vi "Create Transfer Groups.vi"(8 "error in (no error)":errorcluster, 10 "Transfer Group Configurations":T1[](array[typedef]) {"Transfers"."channel configurations"."buffer offset" format="%d bytes"}, 11 "Framework in":refnum<class "Framework.lvclass">) -> (0 "error out":errorcluster, 2 "Transfer Groups":refnum<class "Transfer Group.lvclass">[](array[class]), 3 "Framework out":refnum<class "Framework.lvclass">)   [LabVIEW 2017, in "DSF Core.lvlib" / "Framework.lvclass"]
uses:
  Framework.lvclass
  Transfer Group/Transfer Group.lvclass
  Configuration/Public/Controls/DSF Engine Transfer Group Configuration.ctl
  Configuration/Public/Controls/DSF Direction.ctl
  Configuration/Public/Controls/DSF Timing Info.ctl
  Configuration/Public/Controls/DSF Engine Transfer Configuration.ctl
  Configuration/Public/Controls/DSF Byte Order.ctl
  Configuration/Public/Controls/DSF Engine Channel Configuration.ctl
  Configuration/Public/Controls/DSF Data Type.ctl
  Configuration/Public/Controls/DSF Settings Info.ctl
  Framework.lvclass/Framework.ctl
  Cache/Cache.lvclass/Cache.ctl
  Pointer/DBL Pointer.lvclass
  C:/Program Files (x86)/National Instruments/LabVIEW 2017/vi.lib/NI/Memory Manager/Classes/Pointer/Pointer.lvclass
  <vilib>/NI/Memory Manager/Classes/Pointer/Pointer.lvclass/Pointer.ctl
  <vilib>/NI/Memory Manager/Classes/Pointer/Public/New/New (8B).vi
  <vilib>/NI/Memory Manager/Classes/Pointer/Private/Allocate.vi
  <vilib>/NI/Memory Manager/Classes/Pointer/API/Accessors/Set Address.vi
  <vilib>/NI/Memory Manager/Classes/Pointer/API/Accessors/Set Size.vi
  <vilib>/NI/Memory Manager/Classes/Pointer/Private/Set Internal.vi
  Timing/Timing.lvclass
  Cache/Cache.lvclass
  DSF Core.lvlib
  Buffer/Buffer.lvclass
  <vilib>/NI/Memory Manager/Classes/Pointer/Pointer.lvclass
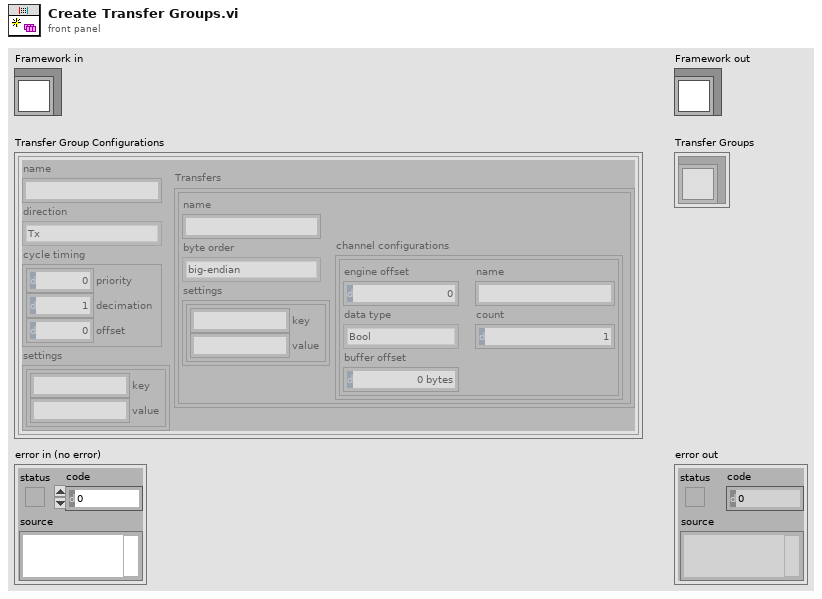
[diagram p1: front panel]
types:
  T1 = typedef "DSF Core.lvlib/DSF Engine Transfer Group Configuration.ctl" = cluster{"name":string, "direction":T2, "cycle timing":T3, "Transfers":T4[], "settings":T8}
  T2 = typedef "DSF Core.lvlib/DSF Direction.ctl" = enum8{"Tx", "Rx"}
  T3 = typedef "DSF Core.lvlib/DSF Timing Info.ctl" = cluster{"priority":u64, "decimation":u64, "offset":u64}
  T4 = typedef "DSF Core.lvlib/DSF Engine Transfer Configuration.ctl" = cluster{"name":string, "byte order":T5, "channel configurations":T6[], "settings":T8}
  T5 = typedef "DSF Core.lvlib/DSF Byte Order.ctl" = enum8{"big-endian", "little-endian"}
  T6 = typedef "DSF Core.lvlib/DSF Engine Channel Configuration.ctl" = cluster{"engine offset":u64, "name":string, "data type":T7, "count":u64, "buffer offset":u64}
  T7 = typedef "DSF Core.lvlib/DSF Data Type.ctl" = enum8{"Bool", "SGL", "DBL", "I8", "I16", "I32", "I64", "U8", "U16", "U32", "U64"}
  T8 = typedef "DSF Core.lvlib/DSF Settings Info.ctl" = cluster{"key":string, "value":string}[]
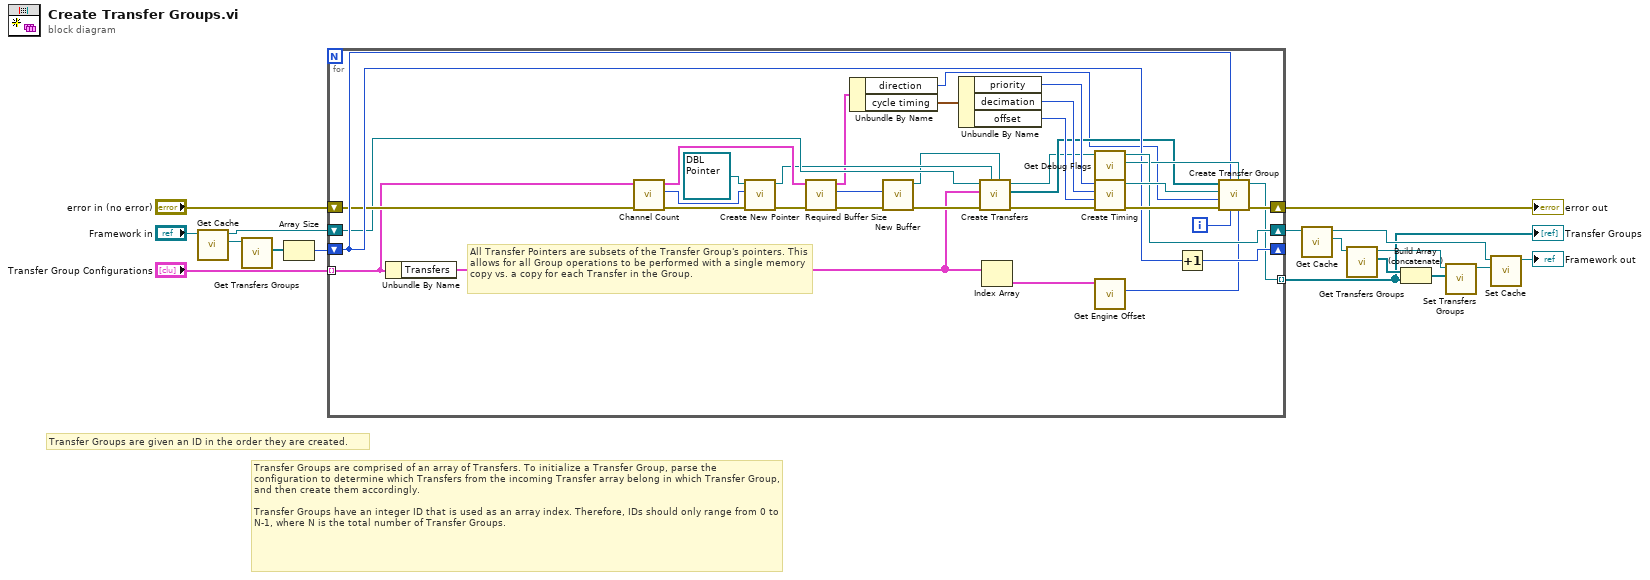
[diagram p0: block diagram]
diagram:
  # "Transfer Groups are given an ID in the order they are created."
  # "Transfer Groups are comprised of an array of Transfers. To initialize a Transfer Group, parse the configuration to determine which Transfers from the incoming Transfer array belong in which Transfer Group, and then create them accordingly.\n\nTransfer Groups have an integer ID that is used as an array index. Therefore, IDs should only range from 0 to N-1, where N is the total number of Transfer Groups."
  n1 = call "Get Cache.vi"("Framework in"="Framework in") -> ("Cache"=w6:refnum<class "Cache.lvclass">, "Framework out"=w4:refnum<class "Framework.lvclass">)  [unwired: 9 in]
  n2 = call "Get Transfers Groups.vi"("Cache in"=w6) -> ("Transfers Groups"=w3:refnum<class "Transfer Group.lvclass">[])  [unwired: 9 in, 1 out]
  n3 = Array Size(array=w3) -> (size(s)=w16:i32)
  n4 = for {
    shift-right: [w51] -> w1
    shift-left: "error in (no error)" -> [w39]
    tunnel: [w40] -> w2 mode=indexing
    shift-right: [w44] -> w8
    shift-left: w4 -> [w31]
    shift-right: [w50] -> _
    shift-left: w16 -> [w42]
    tunnel: "Transfer Group Configurations" -> [w23] mode=indexing
    i -> [w41]
    # "All Transfer Pointers are subsets of the Transfer Group's pointers. This allows for all Group operations to be performed with a single memory copy vs. a copy for each Transfer in the Group."
    n5 = Unbundle By Name(w23) -> ("Transfers"=w22:T4[])
    n6 = call "Channel Count.vi"("error in (no error)"=w39, "Transfer Group Configuration in"=w23) -> ("error out"=w29:errorcluster, "total channel count"=w24:u64, "Transfer Group Configuration out"=w38:T1)  [unwired: 7 in]
    n7 = call-poly <vilib>:"Create New Pointer.vi"("error in (no error)"=w29, "count (1)"=w24, "Pointer type"=refnum<class "DBL Pointer.lvclass"> refnum ("Group Intermediate Buffer")) -> ("error out"=w28:errorcluster, "Pointer"=w27:refnum<class "DBL Pointer.lvclass">)  [unwired: 7 in]
    n8 = call "Required Buffer Size.vi"("error in (no error)"=w28, "Transfer Group Configuration in"=w38) -> ("error out"=w36:errorcluster, "required buffer size"=w37:u64, "Transfer Group Configuration out"=w20:T1)  [unwired: 7 in]
    n9 = Unbundle By Name(w20) -> ("direction"=w19:T2, "cycle timing"=w18:T3)
    n10 = call "New Buffer.vi"("error in (no error)"=w36, "size"=w37) -> ("error out"=w35:errorcluster, "Buffer out"=w26:refnum<class "Buffer.lvclass">)  [unwired: 8 in]
    n11 = Unbundle By Name(w18) -> ("priority"=w46:u64, "decimation"=w47:u64, "offset"=w48:u64)
    n12 = call "Create Transfers.vi"("Group String Buffer"=w26, "Group Intermediate Buffer"=w27, "error in (no error)"=w35, "Transfer Configurations"=w22, "Framework in"=w31) -> ("error out"=w34:errorcluster, "Transfers"=w33:refnum<class "Transfer.lvclass">[], "Framework out"=w32:refnum<class "Framework.lvclass">)  [unwired: 4 in]
    n13 = Index Array(array=w22) -> (element=w21:T4)  [unwired: 1 in]
    n14 = call "Get Debug Flags.vi"("Framework in"=w32) -> ("Debug Flags"=w43:refnum<class "Debug Flags.lvclass">, "Framework out"=w44:refnum<class "Framework.lvclass">)  [unwired: 9 in]
    n15 = call "Create Timing.vi"("error in (no error)"=w34, "Offset"=w48, "Decimation"=w47, "Priority"=w46) -> ("error out"=w49:errorcluster, "Timing"=w45:refnum<class "Timing.lvclass">)  [unwired: 6 in]
    n16 = call "Get Engine Offset.vi"("Transfer Configuration in"=w21) -> ("engine offset"=w25:u64)  [unwired: 9 in, 1 out]
    n17 = Increment(x=w42) -> (x+1=w50:i32)
    n18 = call "Create Transfer Group.vi"("engine offset"=w25, "Debug Flags"=w43, "transceiver id"=w41, "framework id"=w42, "error in (no error)"=w49, "Direction"=w19, "Timing"=w45, "Transfers"=w33) -> ("error out"=w51:errorcluster, "Transfer Group out"=w40:refnum<class "Transfer Group.lvclass">)  [unwired: 2 in]
  }
  "error out" <- w1
  "Transfer Groups" <- w2
  n19 = call "Get Cache.vi"("Framework in"=w8) -> ("Cache"=w13:refnum<class "Cache.lvclass">, "Framework out"=w14:refnum<class "Framework.lvclass">)  [unwired: 9 in]
  n20 = call "Get Transfers Groups.vi"("Cache in"=w13) -> ("Transfers Groups"=w10:refnum<class "Transfer Group.lvclass">[], "Cache out"=w11:refnum<class "Cache.lvclass">)  [unwired: 9 in]
  n21 = Build Array (concatenate)(w10, w2) -> (w9:refnum<class "Transfer Group.lvclass">[])
  n22 = call "Set Transfers Groups.vi"("Transfers Groups"=w9, "Cache in"=w11) -> ("Cache out"=w12:refnum<class "Cache.lvclass">)  [unwired: 9 in]
  n23 = call "Set Cache.vi"("Cache"=w12, "Framework in"=w14) -> ("Framework out"=→"Framework out":refnum<class "Framework.lvclass">)  [unwired: 9 in]
